vi "Build Description String.vi"(8 "error in (no error)":errorcluster, 11 "Keyboard Macro in":refnum<class "Keyboard Macro.lvclass">) -> (0 "error out":errorcluster, 2 "Description":string, 3 "Keyboard Macro out":refnum<class "Keyboard Macro.lvclass">)   [LabVIEW 2020, in "MacroAssert.lvlib" / "Keyboard Macro.lvclass"]
doc: "Builds a string to describe what <B>Step</B> does."
uses:
  Keyboard Macro.lvclass
  Keyboard Macro.lvclass/Keyboard Macro.ctl
  Macro Step/Macro Step.lvclass
panel:
  in  "Virtual Key":u8(ring)=65
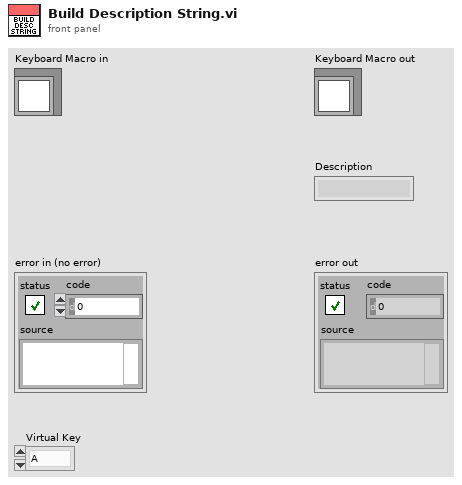
[diagram p1: front panel]
types:
  T1 = typedef "MacroAssert.lvlib/Step Type V3.ctl" = enum16{"Mouse Move", "Mouse Click", "Key Press", "Wait", "Mouse Down", "Mouse Up", "Key Down", "Key Up", "Test Assertion", "Maximize Window", "Restore Window", "Minimize Window", "Close Window", "Bring Window to Front", "Send Window to Back"}
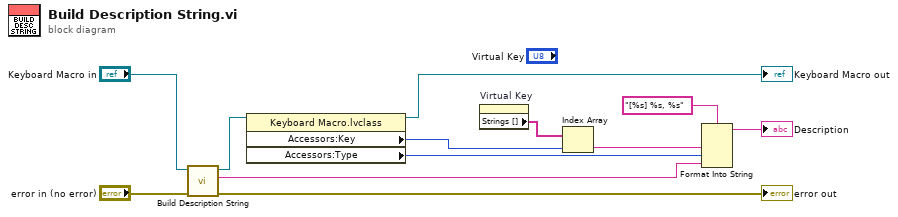
[diagram p0: block diagram]
diagram:
  n1 = call-parent "Build Description String.vi"("error in (no error)"="error in (no error)", "Macro Step in"="Keyboard Macro in") -> ("error out"=→"error out":errorcluster, "Description"=w1:string, "Macro Step out"=w2:refnum<class "Keyboard Macro.lvclass">)  [unwired: 7 in]
  n2 = property class="Keyboard Macro.lvclass"(reference=w2) -> (reference out=→"Keyboard Macro out":refnum<class "Keyboard Macro.lvclass">, "Accessors:Key"=w12:u8, "Accessors:Type"=w5:T1)  [unwired: 1 in, 1 out]
  n3 = property on="Virtual Key" class="Ring (strict)"() -> ("Strings []"=w10:string[])  [unwired: 2 in, 2 out]
  n4 = Index Array(array=w10, index=w12) -> (element=w9:string)
  n5 = Format Into String(format string="[%s] %s, %s", w9, w5, w1) -> (resulting string=→"Description":string)  [unwired: 2 in, 1 out]
